vi "Add Polynomials.vi"   [LabVIEW 2017, in "NI_AALPro.lvlib"]
doc: "Adds two polynomials <B>P(x)</B> and <B>Q(x)</B>. The data types you wire to the <B>P(x)</B> and <B>Q(x)</B> inputs determine the polymorphic instance to use."
uses:
  NI_AALPro.lvlib
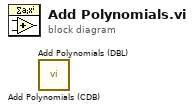
[diagram p0: block diagram]
diagram:
  n1 = call "Add Polynomials (CDB).vi"() -> ()  [unwired: 10 in, 2 out]
  n2 = call "Add Polynomials (DBL).vi"() -> ()  [unwired: 10 in, 2 out]
